vi "PH_AWG-510.ProcCases.vi"(0 "i ref in":refnum<vi>, 1 "selector":string, 2 "Data":T1, 3 "call cluster":T2={"Object"="", "Selector"="", "CallType"=enum."synchronous", "Async Object"="", "Async Selector"="", "Data Descriptor"="", "Data"=[], "Error #"=0, "Expire"=0}, 5 "error in":errorcluster) -> (14 "i ref out":refnum<vi>, 17 "answer cluster":T2={"Object"="", "Selector"="", "CallType"=enum."synchronous", "Async Object"="", "Async Selector"="", "Data Descriptor"="", "Data"=[], "Error #"=0, "Expire"=0}, 19 "error out":errorcluster)   [LabVIEW 2014, in "PH_AWG-510.lvlib"]
doc: "This method is called by a process from within the default case in the event loop. The methods of a class that are linked to events will be called from THIS method. Add your code here."
uses:
  PH_AWG-510.lvlib
  CS_Core/CSSystem/CoreDefs/CoreDefs.call_type.ctl
  CS_Core/BaseProcess/BaseProcess.descriptor string definition.ctl
  CS_Core/CSSystem/CoreDefs/CoreDefs.rawDataType.ctl
  PH_AWG-510.Trigger Settings.ctl
  CS_Core/CSSystem/CoreLib/CoreLib.byte array 2 short.vi
  CS_Core/CSSystem/CoreLib/CoreLib.string 2 byte array.vi
  CS_Core/CSSystem/CoreLib/CoreLib.byte array 2 string.vi
  CS_Core/CSSystem/CoreLib/CoreLib.byte array 2 double.vi
  CS_Core/CSSystem/CoreLib/CoreLib.lvlib
  CS_Core/BaseProcess/BaseProcess.lvlib
  CS_Core/CAEObj/CAEObj.lvlib
  PH_Basics/PH_PSDBWriter/PH_PSDBWriter.lvlib
  instr.lib/awg510/Tektronix AWG510.lvlib
  PH_Basics/PH_Common/PH_Common.lvlib
  PH_Basics/PH_StatusHandler/PH_StatusHandler.lvlib
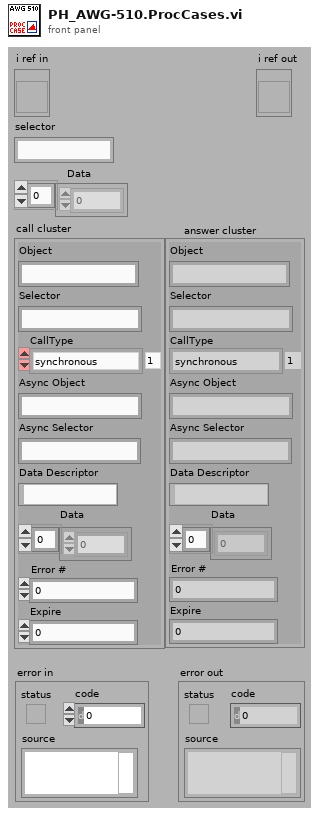
[diagram p1: front panel]
types:
  T1 = typedef "CoreDefs.rawDataType.ctl" = i8[]
  T2 = typedef "CoreDefs.call_type.ctl" = cluster{"Object":string, "Selector":string, "CallType":enum16{"simple", "synchronous", "asynchronous"}, "Async Object":string, "Async Selector":string, "Data Descriptor":T3, "Data":T1, "Error #":i32, "Expire":u32}
  T3 = typedef "BaseProcess.lvlib/BaseProcess.descriptor string definition.ctl" = string
  T4 = typedef "PH_AWG-510.lvlib/PH_AWG-510.Trigger Settings.ctl" = cluster{"Mode":enum16{"Continuous", "Triggered", "Gated", "Enhanced"}, "Level (V)":dbl, "External Source":bool}
  T5 = typedef "PH_AWG-510.lvlib/PH_AWG-510.i attribute.ctl" = cluster{"GUI Refs":cluster{"Delete":refnum<vi>, "Trigger Settings":refnum<vi>, "Start Device":refnum<vi>, "Instrument Information":refnum<vi>, "Lock Frontpanel":refnum<vi>, "Waveform Pattern File":refnum<vi>, "Initialize":refnum<vi>, "Output Settings":refnum<vi>}, "Instrument Information":T6, "Initialized?":bool, "Current Settings":cluster{"Trigger":T4, "Output Settings":T7}, "Wanted Settings":cluster{"Trigger":T4, "Output Settings":T7}, "Device frontpanel locked?":bool, "Default File Path":path}
  T6 = typedef "PH_AWG-510.lvlib/PH_AWG-510.Instrument Information Dataset.ctl" = cluster{"VISA resource name":refnum<visa-resource-name>, "Instrument Firmware Revision":string, "Manufacturer":string, "Model":string, "Serial Number":string, "Error Message":string, "Device Status":enum16{"stopped", "wating for trigger", "running", "Failure"}}
  T7 = typedef "PH_AWG-510.lvlib/PH_AWG-510.Output Settings.ctl" = cluster{"Activate Channel":bool, "VPP (V)":dbl, "Clock (Hz)":dbl, "File Name (Device)":string, "#1":u16, "#2":u16, "#3":u16, "#4":u16, "#5":u16, "#6":u16, "#7":u16, "#8":u16, "#9":u16, "#10":u16, "#11":u16, "#12":u16, "#13":u16, "#14":u16, "#15":u16, "#16":u16, "#17":u16, "#18":u16, "#19":u16, "#20":u16, "Offset (V)":dbl}
  T8 = typedef "PH_PSDBWriter.lvlib/PH_PSDBWriter.PHELIX-Subsystems.ctl" = i32
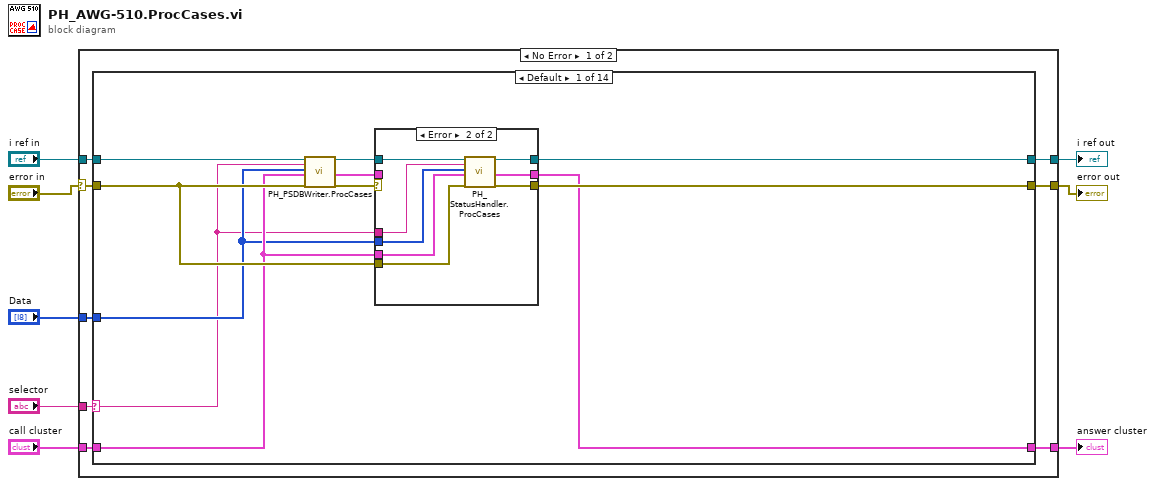
[diagram p0: block diagram]
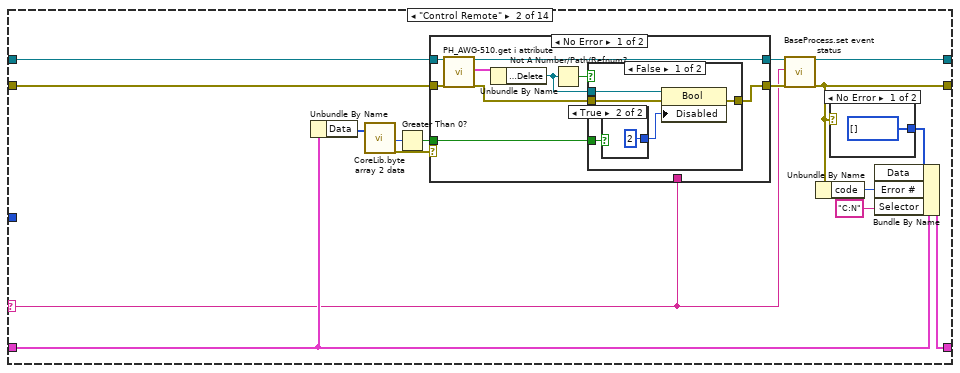
[diagram p3: hidden frame]
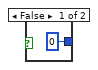
[diagram p4: hidden frame]
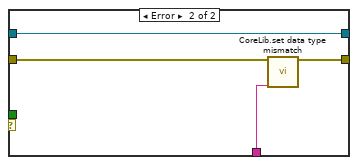
[diagram p6: hidden frame]
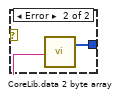
[diagram p7: hidden frame]
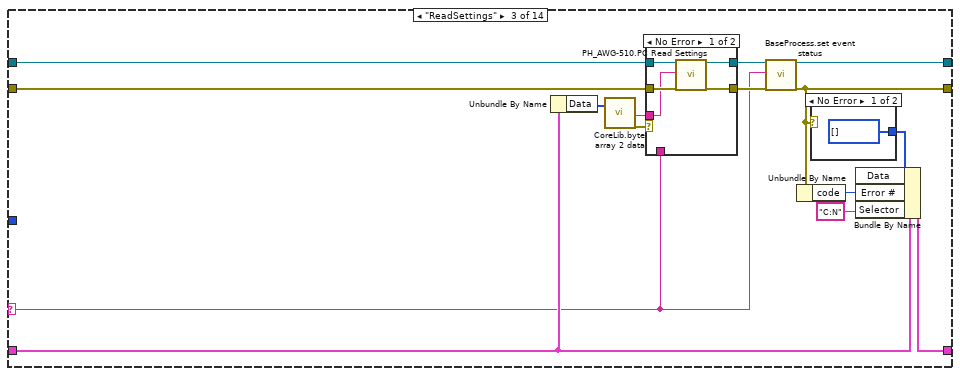
[diagram p8: hidden frame]
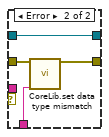
[diagram p9: hidden frame]
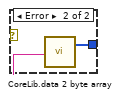
[diagram p10: hidden frame]
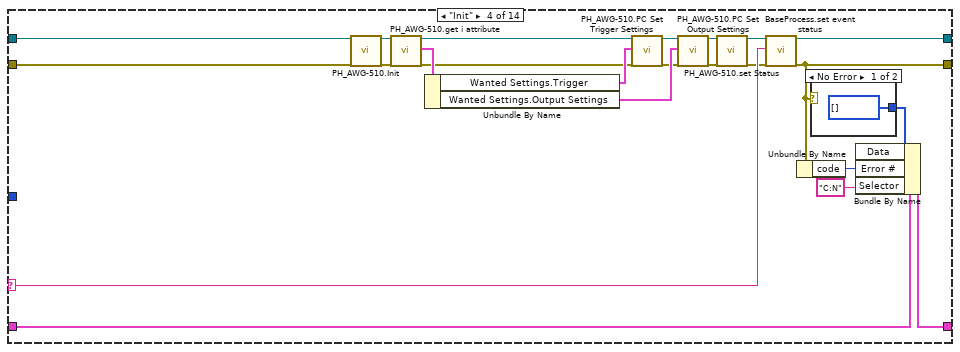
[diagram p11: hidden frame]
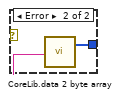
[diagram p12: hidden frame]
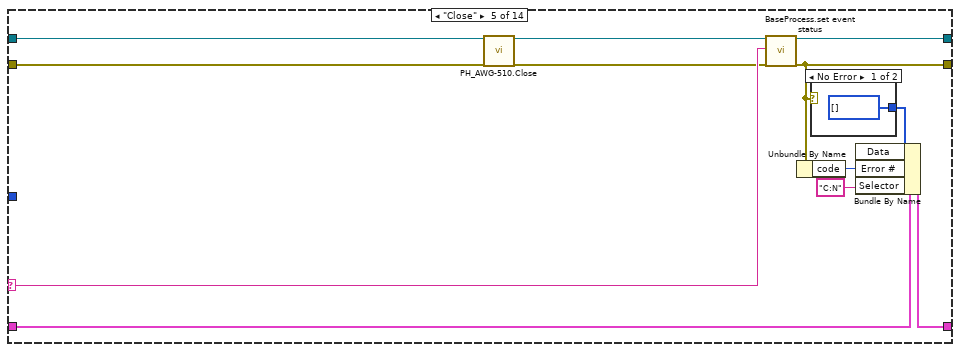
[diagram p13: hidden frame]
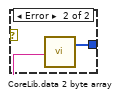
[diagram p14: hidden frame]
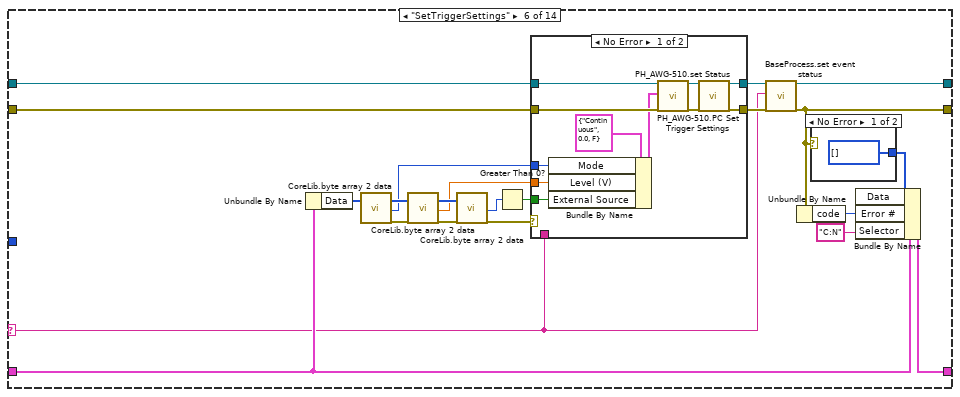
[diagram p15: hidden frame]
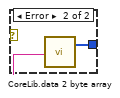
[diagram p17: hidden frame]
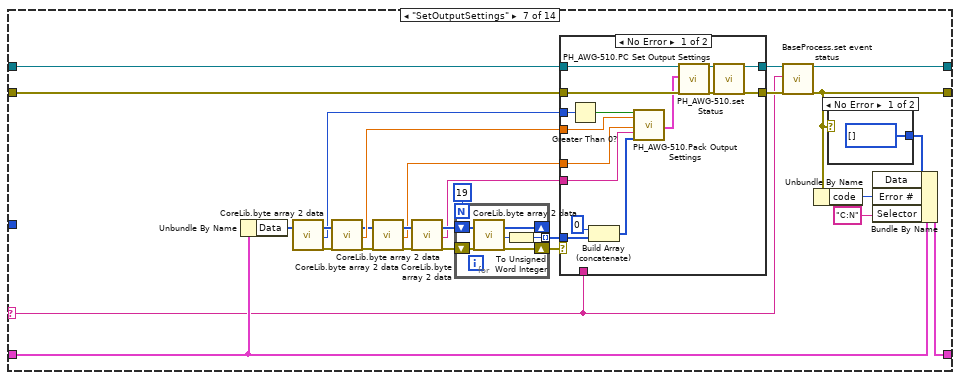
[diagram p18: hidden frame]
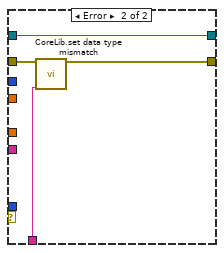
[diagram p19: hidden frame]
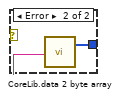
[diagram p20: hidden frame]
diagram:
  n1 = case shown="No Error" "error in" {
    selector: "error in" -> [w9 w513]
    tunnel: "selector" -> [w16 _]
    tunnel: [w15 w514] -> w7
    tunnel: "call cluster" -> [w14 w514]
    tunnel: "i ref in" -> [w13 w515]
    tunnel: [w12 w515] -> w4
    tunnel: [w11 w513] -> w3
    tunnel: "Data" -> [w10 _]
    frame No Error {
      n2 = case shown="Default" w16 {
        selector: w16 -> [w19 w39 w81 w123 w139 w158 w208 w252 w309 w355 w384 w435 w453 w470]
        tunnel: w13 -> [w27 w43 w87 w122 w138 w162 w212 w256 w313 w359 w388 w439 w457 w472]
        tunnel: [w24 w51 w91 w127 w143 w169 w216 w260 w317 w363 w392 w443 w461 w483] -> w12
        tunnel: w14 -> [w21 w40 w83 w124 w140 w159 w209 w253 w310 w356 w385 w436 w454 w480]
        tunnel: [w23 w49 w89 w125 w141 w167 w214 w258 w315 w361 w390 w441 w459 w481] -> w15
        tunnel: w9 -> [w22 w44 w88 w121 w136 w163 w213 w257 w314 w360 w389 w440 w458 w471]
        tunnel: [w26 w50 w90 w126 w142 w168 w215 w259 w316 w362 w391 w442 w460 w482] -> w11
        tunnel: w10 -> [w20 _ _ _ _ _ _ _ _ _ _ _ _ w469]
        frame Default {
          # "In the default case, always call the ProcCase method of the parent class"
          n3 = call "PH_PSDBWriter.ProcCases.vi"("i ref in"=w27, "selector"=w19, "Data"=w20, "call cluster"=w21, "error in"=w22) -> ("i ref out"=w25:refnum<vi>, "answer cluster"=w17:T2, "error out"=w18:errorcluster)  [unwired: 12 in]
          n4 = case shown="Error" w18 {
            selector: w18 -> [w28 _]
            tunnel: [w28 w38] -> w26
            tunnel: w25 -> [w30 w37]
            tunnel: [w30 w36] -> w24
            tunnel: [w29 w35] -> w23
            tunnel: w22 -> [_ w34]
            tunnel: w21 -> [_ w33]
            tunnel: w20 -> [_ w32]
            tunnel: w19 -> [_ w31]
            tunnel: w17 -> [w29 _]
            frame No Error {
            }
            frame Error {
              n5 = call "PH_StatusHandler.ProcCases.vi"("i ref in"=w37, "selector"=w31, "Data"=w32, "call cluster"=w33, "error in (no error)"=w34) -> ("i ref out"=w36:refnum<vi>, "answer cluster"=w35:T2, "error out"=w38:errorcluster)  [unwired: 12 in]
            }
          }
        }
        frame "Control Remote" {
          n6 = Unbundle By Name(w40) -> ("Data"=w45:T1)
          n7 = call-poly "CoreLib.byte array 2 data.vi"("byteArray"=w45) -> ("i16"=w46:i16, "error out"=w48:errorcluster)  [unwired: 16 in, 1 out]
          n8 = Greater Than 0?(x=w46) -> (x > 0?=w47:bool)
          n9 = case shown="No Error" w48 {
            tunnel: [w57 w75] -> w42
            tunnel: w43 -> [w63 w75]
            tunnel: w44 -> [w62 w74]
            tunnel: [w58 w73] -> w41
            tunnel: w39 -> [_ w72]
            tunnel: w47 -> [w59 _]
            frame No Error {
              n10 = call "PH_AWG-510.get i attribute.vi"("i ref in"=w63, "error in (no error)"=w62) -> ("i ref out"=w57:refnum<vi>, "i attribute"=w61:T5, "error out"=w60:errorcluster)  [unwired: 15 in]
              n11 = Unbundle By Name(w61) -> ("GUI Refs.Delete"=w56:refnum<vi>)
              n12 = Not A Number/Path/Refnum?(number/path/refnum=w56) -> (NaN/Path/Refnum?=w55:bool)
              n13 = case shown="False" w55 {
                tunnel: w56 -> [w68 _]
                tunnel: w60 -> [w67 w71]
                tunnel: [w66 w71] -> w58
                tunnel: w59 -> [w65 _]
                frame False {
                  n14 = case shown="True" w65 {
                    tunnel: [0 2] -> w64
                    frame False {
                    }
                    frame True {
                    }
                  }
                  n15 = property class="Bool"(reference=w68, error in=w67, "Disabled"=w64) -> (error out=w66:errorcluster)  [unwired: 1 out]
                }
                frame True {
                }
              }
            }
            frame Error {
              n16 = call "CoreLib.set data type mismatch.vi"("error in (no error)"=w74, "error source"=w72) -> ("error out"=w73:errorcluster)  [unwired: 17 in]
            }
          }
          n17 = call "BaseProcess.set event status.vi"("i ref in"=w42, "EventStatus"=w39, "error in (no error)"=w41) -> ("i ref out"=w51:refnum<vi>, "error out"=w50:errorcluster)  [unwired: 14 in, 1 out]
          n18 = Unbundle By Name(w50) -> ("code"=w54:i32)
          n19 = case shown="No Error" w50 {
            selector: w50 -> [_ w79]
            tunnel: [T1 [] ("byteArray out") w77] -> w53
            frame No Error {
            }
            frame Error {
              n20 = Unbundle By Name(w79) -> ("source"=w78:string)
              n21 = call-poly "CoreLib.data 2 byte array.vi"("string"=w78) -> ("byteArray out"=w77:T1)  [unwired: 18 in]
            }
          }
          n22 = Bundle By Name(cluster=w40, "Data"=w53, "Error #"=w54, "Selector"="C:N") -> (w49:T2)
        }
        frame "ReadSettings" {
          n23 = Unbundle By Name(w83) -> ("Data"=w84:T1)
          n24 = call-poly "CoreLib.byte array 2 data.vi"("byteArray"=w84) -> ("string"=w80:string, "error out"=w82:errorcluster)  [unwired: 16 in, 1 out]
          n25 = case shown="No Error" w82 {
            tunnel: w88 -> [w96 w102]
            tunnel: w87 -> [w99 w100]
            tunnel: [w98 w100] -> w86
            tunnel: [w97 w101] -> w85
            tunnel: w80 -> [w95 _]
            tunnel: w81 -> [_ w103]
            frame No Error {
              n26 = call "PH_AWG-510.PC Read Settings.vi"("VI in"=w99, "File"=w95, "error in (no error)"=w96) -> ("VI out"=w98:refnum<vi>, "error out"=w97:errorcluster)  [unwired: 15 in]
            }
            frame Error {
              n27 = call "CoreLib.set data type mismatch.vi"("error in (no error)"=w102, "error source"=w103) -> ("error out"=w101:errorcluster)  [unwired: 17 in]
            }
          }
          n28 = call "BaseProcess.set event status.vi"("i ref in"=w86, "EventStatus"=w81, "error in (no error)"=w85) -> ("i ref out"=w91:refnum<vi>, "error out"=w90:errorcluster)  [unwired: 14 in, 1 out]
          n29 = Unbundle By Name(w90) -> ("code"=w94:i32)
          n30 = case shown="No Error" w90 {
            selector: w90 -> [_ w107]
            tunnel: [T1 [] ("byteArray out") w105] -> w93
            frame No Error {
            }
            frame Error {
              n31 = Unbundle By Name(w107) -> ("source"=w106:string)
              n32 = call-poly "CoreLib.data 2 byte array.vi"("string"=w106) -> ("byteArray out"=w105:T1)  [unwired: 18 in]
            }
          }
          n33 = Bundle By Name(cluster=w83, "Data"=w93, "Error #"=w94, "Selector"="C:N") -> (w89:T2)
        }
        frame "Init" {
          n34 = call "PH_AWG-510.Init.vi"("VI in"=w122, "error in (no error)"=w121) -> ("VI out"=w111:refnum<vi>, "error out"=w109:errorcluster)  [unwired: 16 in]
          n35 = call "PH_AWG-510.get i attribute.vi"("i ref in"=w111, "error in (no error)"=w109) -> ("i ref out"=w114:refnum<vi>, "i attribute"=w115:T5, "error out"=w112:errorcluster)  [unwired: 15 in]
          n36 = Unbundle By Name(w115) -> ("Wanted Settings.Trigger"=w116:T4, "Wanted Settings.Output Settings"=w118:T7)
          n37 = call "PH_AWG-510.PC Set Trigger Settings.vi"("VI in"=w114, "Wanted Trigger Settings"=w116, "error in (no error)"=w112) -> ("VI out"=w117:refnum<vi>, "error out"=w113:errorcluster)  [unwired: 15 in]
          n38 = call "PH_AWG-510.PC Set Output Settings.vi"("VI in"=w117, "Wanted Output Settings"=w118, "error in (no error)"=w113) -> ("VI out"=w110:refnum<vi>, "error out"=w108:errorcluster)  [unwired: 15 in]
          n39 = call "PH_AWG-510.set Status.vi"("i ref in"=w110, "error in"=w108) -> ("i ref out"=w120:refnum<vi>, "error out"=w119:errorcluster)  [unwired: 16 in]
          n40 = call "BaseProcess.set event status.vi"("i ref in"=w120, "EventStatus"=w123, "error in (no error)"=w119) -> ("i ref out"=w127:refnum<vi>, "error out"=w126:errorcluster)  [unwired: 14 in, 1 out]
          n41 = Unbundle By Name(w126) -> ("code"=w130:i32)
          n42 = case shown="No Error" w126 {
            selector: w126 -> [_ w134]
            tunnel: [T1 [] ("byteArray out") w132] -> w129
            frame No Error {
            }
            frame Error {
              n43 = Unbundle By Name(w134) -> ("source"=w133:string)
              n44 = call-poly "CoreLib.data 2 byte array.vi"("string"=w133) -> ("byteArray out"=w132:T1)  [unwired: 18 in]
            }
          }
          n45 = Bundle By Name(cluster=w124, "Data"=w129, "Error #"=w130, "Selector"="C:N") -> (w125:T2)
        }
        frame "Close" {
          n46 = call "PH_AWG-510.Close.vi"("VI in"=w138, "error in (no error)"=w136) -> ("VI out"=w137:refnum<vi>, "error out"=w135:errorcluster)  [unwired: 16 in]
          n47 = call "BaseProcess.set event status.vi"("i ref in"=w137, "EventStatus"=w139, "error in (no error)"=w135) -> ("i ref out"=w143:refnum<vi>, "error out"=w142:errorcluster)  [unwired: 14 in, 1 out]
          n48 = Unbundle By Name(w142) -> ("code"=w146:i32)
          n49 = case shown="No Error" w142 {
            selector: w142 -> [_ w150]
            tunnel: [T1 [] ("byteArray out") w148] -> w145
            frame No Error {
            }
            frame Error {
              n50 = Unbundle By Name(w150) -> ("source"=w149:string)
              n51 = call-poly "CoreLib.data 2 byte array.vi"("string"=w149) -> ("byteArray out"=w148:T1)  [unwired: 18 in]
            }
          }
          n52 = Bundle By Name(cluster=w140, "Data"=w145, "Error #"=w146, "Selector"="C:N") -> (w141:T2)
        }
        frame "SetTriggerSettings" {
          n53 = Unbundle By Name(w159) -> ("Data"=w156:T1)
          n54 = call-poly "CoreLib.byte array 2 data.vi"("byteArray"=w156) -> ("byteArray out"=w157:T1, "i16"=w152:i16, "error out"=w154:errorcluster)  [unwired: 16 in]
          n55 = call-poly "CoreLib.byte array 2 data.vi"("byteArray"=w157, "error in (no error)"=w154) -> ("byteArray out"=w155:T1, "d64"=w151:dbl, "error out"=w153:errorcluster)  [unwired: 15 in]
          n56 = call-poly "CoreLib.byte array 2 data.vi"("byteArray"=w155, "error in (no error)"=w153) -> ("i16"=w164:i16, "error out"=w166:errorcluster)  [unwired: 15 in, 1 out]
          n57 = Greater Than 0?(x=w164) -> (x > 0?=w165:bool)
          n58 = case shown="No Error" w166 {
            tunnel: [w175 w187] -> w161
            tunnel: w162 -> [w183 w187]
            tunnel: w163 -> [w182 w186]
            tunnel: [w173 w185] -> w160
            tunnel: w158 -> [_ w184]
            tunnel: w165 -> [w178 _]
            tunnel: w152 -> [w180 _]
            tunnel: w151 -> [w179 _]
            frame No Error {
              n59 = Bundle By Name(cluster=T4 {"Mode"=enum."Continuous", "Level (V)"=0.0, "External Source"=FALSE} ("Wanted Trigger Settings"), "Mode"=w180, "Level (V)"=w179, "External Source"=w178) -> (w177:T4)
              n60 = call "PH_AWG-510.PC Set Trigger Settings.vi"("VI in"=w183, "Wanted Trigger Settings"=w177, "error in (no error)"=w182) -> ("VI out"=w176:refnum<vi>, "error out"=w174:errorcluster)  [unwired: 15 in]
              n61 = call "PH_AWG-510.set Status.vi"("i ref in"=w176, "error in"=w174) -> ("i ref out"=w175:refnum<vi>, "error out"=w173:errorcluster)  [unwired: 16 in]
            }
            frame Error {
              n62 = call "CoreLib.set data type mismatch.vi"("error in (no error)"=w186, "error source"=w184) -> ("error out"=w185:errorcluster)  [unwired: 17 in]
            }
          }
          n63 = call "BaseProcess.set event status.vi"("i ref in"=w161, "EventStatus"=w158, "error in (no error)"=w160) -> ("i ref out"=w169:refnum<vi>, "error out"=w168:errorcluster)  [unwired: 14 in, 1 out]
          n64 = Unbundle By Name(w168) -> ("code"=w172:i32)
          n65 = case shown="No Error" w168 {
            selector: w168 -> [_ w191]
            tunnel: [T1 [] ("byteArray out") w189] -> w171
            frame No Error {
            }
            frame Error {
              n66 = Unbundle By Name(w191) -> ("source"=w190:string)
              n67 = call-poly "CoreLib.data 2 byte array.vi"("string"=w190) -> ("byteArray out"=w189:T1)  [unwired: 18 in]
            }
          }
          n68 = Bundle By Name(cluster=w159, "Data"=w171, "Error #"=w172, "Selector"="C:N") -> (w167:T2)
        }
        frame "SetOutputSettings" {
          n69 = Unbundle By Name(w209) -> ("Data"=w206:T1)
          n70 = call-poly "CoreLib.byte array 2 data.vi"("byteArray"=w206) -> ("byteArray out"=w207:T1, "i16"=w204:i16, "error out"=w205:errorcluster)  [unwired: 16 in]
          n71 = call-poly "CoreLib.byte array 2 data.vi"("byteArray"=w207, "error in (no error)"=w205) -> ("byteArray out"=w193:T1, "d64"=w203:dbl, "error out"=w192:errorcluster)  [unwired: 15 in]
          n72 = call-poly "CoreLib.byte array 2 data.vi"("byteArray"=w193, "error in (no error)"=w192) -> ("byteArray out"=w201:T1, "d64"=w200:dbl, "error out"=w202:errorcluster)  [unwired: 15 in]
          n73 = call-poly "CoreLib.byte array 2 data.vi"("byteArray"=w201, "error in (no error)"=w202) -> ("byteArray out"=w198:T1, "string"=w196:string, "error out"=w199:errorcluster)  [unwired: 15 in]
          n74 = for {
            N: 19 -> [_]
            tunnel: [w220] -> w197 mode=indexing
            shift-right: [w222] -> w195
            shift-left: w199 -> [w225]
            shift-right: [w221] -> _
            shift-left: w198 -> [w224]
            n75 = call-poly "CoreLib.byte array 2 data.vi"("byteArray"=w224, "error in (no error)"=w225) -> ("byteArray out"=w221:T1, "i16"=w223:i16, "error out"=w222:errorcluster)  [unwired: 15 in]
            n76 = To Unsigned Word Integer(number=w223) -> (unsigned 16bit integer=w220:u16)
          }
          n77 = case shown="No Error" w195 {
            tunnel: [w234 w244] -> w211
            tunnel: w212 -> [w240 w244]
            tunnel: w213 -> [w239 w243]
            tunnel: [w232 w242] -> w210
            tunnel: w208 -> [_ w241]
            tunnel: w196 -> [w229 _]
            tunnel: w204 -> [w238 _]
            tunnel: w203 -> [w237 _]
            tunnel: w200 -> [w230 _]
            tunnel: w197 -> [w228 _]
            frame No Error {
              n78 = Greater Than 0?(x=w238) -> (x > 0?=w231:bool)
              n79 = Build Array (concatenate)(u16 0, w228) -> (w227:u16[])
              n80 = call "PH_AWG-510.Pack Output Settings.vi"("Activate Channel"=w231, "VPP [Volts]"=w237, "Clock [Hz]"=w230, "File Name"=w229, "Waveform Pattern [#1 ... #20]"=w227) -> ("Output Settings"=w236:T7)  [unwired: 14 in]
              n81 = call "PH_AWG-510.PC Set Output Settings.vi"("VI in"=w240, "Wanted Output Settings"=w236, "error in (no error)"=w239) -> ("VI out"=w235:refnum<vi>, "error out"=w233:errorcluster)  [unwired: 15 in]
              n82 = call "PH_AWG-510.set Status.vi"("i ref in"=w235, "error in"=w233) -> ("i ref out"=w234:refnum<vi>, "error out"=w232:errorcluster)  [unwired: 16 in]
            }
            frame Error {
              n83 = call "CoreLib.set data type mismatch.vi"("error in (no error)"=w243, "error source"=w241) -> ("error out"=w242:errorcluster)  [unwired: 17 in]
            }
          }
          n84 = call "BaseProcess.set event status.vi"("i ref in"=w211, "EventStatus"=w208, "error in (no error)"=w210) -> ("i ref out"=w216:refnum<vi>, "error out"=w215:errorcluster)  [unwired: 14 in, 1 out]
          n85 = Unbundle By Name(w215) -> ("code"=w219:i32)
          n86 = case shown="No Error" w215 {
            selector: w215 -> [_ w248]
            tunnel: [T1 [] ("byteArray out") w246] -> w218
            frame No Error {
            }
            frame Error {
              n87 = Unbundle By Name(w248) -> ("source"=w247:string)
              n88 = call-poly "CoreLib.data 2 byte array.vi"("string"=w247) -> ("byteArray out"=w246:T1)  [unwired: 18 in]
            }
          }
          n89 = Bundle By Name(cluster=w209, "Data"=w218, "Error #"=w219, "Selector"="C:N") -> (w214:T2)
        }
        frame "SetWfmFile" {
          n90 = Unbundle By Name(w253) -> ("Data"=w249:T1)
          n91 = call-poly "CoreLib.byte array 2 data.vi"("byteArray"=w249) -> ("string"=w250:string, "error out"=w251:errorcluster)  [unwired: 16 in, 1 out]
          n92 = case shown="No Error" w251 {
            tunnel: [w272 w301] -> w255
            tunnel: w256 -> [w269 w301]
            tunnel: w257 -> [w270 w300]
            tunnel: [w271 w299] -> w254
            tunnel: w252 -> [_ w298]
            tunnel: w250 -> [w264 _]
            frame No Error {
              n93 = case shown="Default" w264 {
                selector: w264 -> [_ w275]
                tunnel: w270 -> [w273 w283]
                tunnel: w269 -> [w274 w282]
                tunnel: [w273 w280] -> w268
                tunnel: [w274 w276] -> w266
                frame "", "N/A" {
                }
                frame Default {
                  n94 = call "PH_AWG-510.get data to modify.vi"("i ref in"=w282, "error in (no error)"=w283) -> ("i ref out"=w281:refnum<vi>, "i attribute"=w277:T5, "timed out"=w278:bool, "error out"=w279:errorcluster)  [unwired: 14 in]
                  n95 = case shown="False" w278 {
                    tunnel: w281 -> [w292 w297]
                    tunnel: [w291 w297] -> w276
                    tunnel: [w290 w296] -> w280
                    tunnel: w275 -> [w284 _]
                    tunnel: w279 -> [w289 w296]
                    tunnel: w277 -> [w288 _]
                    frame False {
                      n96 = Unbundle By Name(w288) -> ("Initialized?"=w286:bool, "Instrument Information.VISA resource name"=w287:refnum<visa-resource-name>)
                      n97 = Bundle By Name(cluster=w288, "Current Settings.Output Settings.File Name (Device)"=w284, "Wanted Settings.Output Settings.File Name (Device)"=w284) -> (w285:T5)
                      n98 = case shown="True" w286 {
                        tunnel: w284 -> [_ w295]
                        tunnel: w289 -> [_ w294]
                        tunnel: w287 -> [_ w293]
                        frame False {
                        }
                        frame True {
                          n99 = call "SelectWfmFile.vi"("VISA resource name"=w293, "File name"=w295, "error in"=w294) -> ()  [unwired: 15 in, 2 out]
                        }
                      }
                      n100 = call "PH_AWG-510.set modified data.vi"("i ref in"=w292, "i attribute"=w285, "error in (no error)"=w289) -> ("i ref out"=w291:refnum<vi>, "error out"=w290:errorcluster)  [unwired: 15 in]
                    }
                    frame True {
                    }
                  }
                }
              }
              n101 = call "PH_AWG-510.PC Get Output Settings.vi"("VI in"=w266, "error in (no error)"=w268) -> ("VI out"=w265:refnum<vi>, "error out"=w267:errorcluster)  [unwired: 16 in]
              n102 = call "PH_AWG-510.set Status.vi"("i ref in"=w265, "error in"=w267) -> ("i ref out"=w272:refnum<vi>, "error out"=w271:errorcluster)  [unwired: 16 in]
            }
            frame Error {
              n103 = call "CoreLib.set data type mismatch.vi"("error in (no error)"=w300, "error source"=w298) -> ("error out"=w299:errorcluster)  [unwired: 17 in]
            }
          }
          n104 = call "BaseProcess.set event status.vi"("i ref in"=w255, "EventStatus"=w252, "error in (no error)"=w254) -> ("i ref out"=w260:refnum<vi>, "error out"=w259:errorcluster)  [unwired: 14 in, 1 out]
          n105 = Unbundle By Name(w259) -> ("code"=w263:i32)
          n106 = case shown="No Error" w259 {
            selector: w259 -> [_ w305]
            tunnel: [T1 [] ("byteArray out") w303] -> w262
            frame No Error {
            }
            frame Error {
              n107 = Unbundle By Name(w305) -> ("source"=w304:string)
              n108 = call-poly "CoreLib.data 2 byte array.vi"("string"=w304) -> ("byteArray out"=w303:T1)  [unwired: 18 in]
            }
          }
          n109 = Bundle By Name(cluster=w253, "Data"=w262, "Error #"=w263, "Selector"="C:N") -> (w258:T2)
        }
        frame "StartDevice" {
          n110 = Unbundle By Name(w310) -> ("Data"=w306:T1)
          n111 = call-poly "CoreLib.byte array 2 data.vi"("byteArray"=w306) -> ("i16"=w307:i16, "error out"=w308:errorcluster)  [unwired: 16 in, 1 out]
          n112 = case shown="No Error" w308 {
            tunnel: [w321 w347] -> w312
            tunnel: w313 -> [w326 w347]
            tunnel: w314 -> [w327 w346]
            tunnel: [w322 w345] -> w311
            tunnel: w309 -> [_ w344]
            tunnel: w307 -> [w325 _]
            frame No Error {
              n113 = flat-sequence {
                tunnel: w327 -> [w336]
                tunnel: w326 -> [w335]
                tunnel: w325 -> [w334]
                tunnel: [w333] -> w324
                tunnel: [w332] -> w323
                tunnel: [w340] -> w322
                tunnel: [w342] -> w321
                tunnel: w324 -> [w343]
                tunnel: w323 -> [w341]
                frame #0 {
                  n114 = call "PH_AWG-510.get i attribute.vi"("i ref in"=w335, "error in (no error)"=w336) -> ("i ref out"=w333:refnum<vi>, "i attribute"=w330:T5, "error out"=w332:errorcluster)  [unwired: 15 in]
                  n115 = Greater Than 0?(x=w334) -> (x > 0?=w331:bool)
                  n116 = Unbundle By Name(w330) -> ("Initialized?"=w328:bool, "Instrument Information.VISA resource name"=w329:refnum<visa-resource-name>)
                  n117 = case shown="True" w328 {
                    tunnel: w331 -> [_ w338]
                    tunnel: w332 -> [_ w339]
                    tunnel: w329 -> [_ w337]
                    frame False {
                    }
                    frame True {
                      n118 = call "SetRun.vi"("VISA resource name"=w337, "State"=w338, "error in"=w339) -> ()  [unwired: 15 in, 2 out]
                    }
                  }
                }
                frame #1 {
                  n119 = call "PH_AWG-510.set Status.vi"("i ref in"=w343, "error in"=w341) -> ("i ref out"=w342:refnum<vi>, "error out"=w340:errorcluster)  [unwired: 16 in]
                }
              }
            }
            frame Error {
              n120 = call "CoreLib.set data type mismatch.vi"("error in (no error)"=w346, "error source"=w344) -> ("error out"=w345:errorcluster)  [unwired: 17 in]
            }
          }
          n121 = call "BaseProcess.set event status.vi"("i ref in"=w312, "EventStatus"=w309, "error in (no error)"=w311) -> ("i ref out"=w317:refnum<vi>, "error out"=w316:errorcluster)  [unwired: 14 in, 1 out]
          n122 = Unbundle By Name(w316) -> ("code"=w320:i32)
          n123 = case shown="No Error" w316 {
            selector: w316 -> [_ w351]
            tunnel: [T1 [] ("byteArray out") w349] -> w319
            frame No Error {
            }
            frame Error {
              n124 = Unbundle By Name(w351) -> ("source"=w350:string)
              n125 = call-poly "CoreLib.data 2 byte array.vi"("string"=w350) -> ("byteArray out"=w349:T1)  [unwired: 18 in]
            }
          }
          n126 = Bundle By Name(cluster=w310, "Data"=w319, "Error #"=w320, "Selector"="C:N") -> (w315:T2)
        }
        frame "SetExpMode" {
          n127 = Unbundle By Name(w356) -> ("Data"=w352:T1)
          n128 = call-poly "CoreLib.byte array 2 data.vi"("byteArray"=w352) -> ("i16"=w353:i16, "error out"=w354:errorcluster)  [unwired: 16 in, 1 out]
          n129 = case shown="Error" w354 {
            tunnel: [w370 w376] -> w358
            tunnel: w359 -> [w368 w376]
            tunnel: w360 -> [w369 w375]
            tunnel: [w371 w374] -> w357
            tunnel: w355 -> [_ w373]
            tunnel: w353 -> [w372 _]
            frame No Error {
              n130 = Greater Than 0?(x=w372) -> (x > 0?=w367:bool)
              n131 = call "PH_AWG-510.PC Set Expert Mode.vi"("VI in"=w368, "Expert Mode"=w367, "error in (no error)"=w369) -> ("VI out"=w370:refnum<vi>, "error out"=w371:errorcluster)  [unwired: 15 in]
            }
            frame Error {
              n132 = call "CoreLib.set data type mismatch.vi"("error in (no error)"=w375, "error source"=w373) -> ("error out"=w374:errorcluster)  [unwired: 17 in]
            }
          }
          n133 = call "BaseProcess.set event status.vi"("i ref in"=w358, "EventStatus"=w355, "error in (no error)"=w357) -> ("i ref out"=w363:refnum<vi>, "error out"=w362:errorcluster)  [unwired: 14 in, 1 out]
          n134 = Unbundle By Name(w362) -> ("code"=w366:i32)
          n135 = case shown="No Error" w362 {
            selector: w362 -> [_ w380]
            tunnel: [T1 [] ("byteArray out") w378] -> w365
            frame No Error {
            }
            frame Error {
              n136 = Unbundle By Name(w380) -> ("source"=w379:string)
              n137 = call-poly "CoreLib.data 2 byte array.vi"("string"=w379) -> ("byteArray out"=w378:T1)  [unwired: 18 in]
            }
          }
          n138 = Bundle By Name(cluster=w356, "Data"=w365, "Error #"=w366, "Selector"="C:N") -> (w361:T2)
        }
        frame "LockDevice" {
          n139 = Unbundle By Name(w385) -> ("Data"=w381:T1)
          n140 = call-poly "CoreLib.byte array 2 data.vi"("byteArray"=w381) -> ("i16"=w382:i16, "error out"=w383:errorcluster)  [unwired: 16 in, 1 out]
          n141 = case shown="No Error" w383 {
            tunnel: [w402 w428] -> w387
            tunnel: w388 -> [w406 w428]
            tunnel: w389 -> [w407 w427]
            tunnel: [w403 w426] -> w386
            tunnel: w384 -> [_ w425]
            tunnel: w382 -> [w405 _]
            frame No Error {
              n142 = Greater Than 0?(x=w405) -> (x > 0?=w397:bool)
              n143 = call "PH_AWG-510.get data to modify.vi"("i ref in"=w406, "error in (no error)"=w407) -> ("i ref out"=w400:refnum<vi>, "i attribute"=w398:T5, "timed out"=w396:bool, "error out"=w404:errorcluster)  [unwired: 14 in]
              n144 = case shown="False" w396 {
                tunnel: w404 -> [w419 w423]
                tunnel: [w417 w423] -> w401
                tunnel: w400 -> [w416 w424]
                tunnel: [w415 w424] -> w399
                tunnel: w398 -> [w414 _]
                tunnel: w397 -> [w410 _]
                frame False {
                  n145 = Unbundle By Name(w414) -> ("GUI Refs.Lock Frontpanel"=w411:refnum<vi>, "Initialized?"=w409:bool, "Instrument Information.VISA resource name"=w418:refnum<visa-resource-name>)
                  n146 = Select(t=w410, s=w409, f=w409) -> (s? t:f=w408:bool)
                  n147 = Bundle By Name(cluster=w414, "Device frontpanel locked?"=w408) -> (w413:T5)
                  n148 = call "PH_GUI.set boolean GUI object.vi"("Boolean Knob GUI Ref"=w411, "Value"=w408, "error in (no error)"=w419) -> ("error out"=w412:errorcluster)  [unwired: 16 in]
                  n149 = case shown="True" w409 {
                    tunnel: w410 -> [_ w421]
                    tunnel: w419 -> [_ w422]
                    tunnel: w418 -> [_ w420]
                    frame False {
                    }
                    frame True {
                      n150 = call "SetPanelLock.vi"("VISA resource name"=w420, "Status (Lock)"=w421, "error in"=w422) -> ()  [unwired: 15 in, 2 out]
                    }
                  }
                  n151 = call "PH_AWG-510.set modified data.vi"("i ref in"=w416, "i attribute"=w413, "error in (no error)"=w412) -> ("i ref out"=w415:refnum<vi>, "error out"=w417:errorcluster)  [unwired: 15 in]
                }
                frame True {
                }
              }
              n152 = call "PH_AWG-510.set Status.vi"("i ref in"=w399, "error in"=w401) -> ("i ref out"=w402:refnum<vi>, "error out"=w403:errorcluster)  [unwired: 16 in]
            }
            frame Error {
              n153 = call "CoreLib.set data type mismatch.vi"("error in (no error)"=w427, "error source"=w425) -> ("error out"=w426:errorcluster)  [unwired: 17 in]
            }
          }
          n154 = call "BaseProcess.set event status.vi"("i ref in"=w387, "EventStatus"=w384, "error in (no error)"=w386) -> ("i ref out"=w392:refnum<vi>, "error out"=w391:errorcluster)  [unwired: 14 in, 1 out]
          n155 = Unbundle By Name(w391) -> ("code"=w395:i32)
          n156 = case shown="No Error" w391 {
            selector: w391 -> [_ w432]
            tunnel: [T1 [] ("byteArray out") w430] -> w394
            frame No Error {
            }
            frame Error {
              n157 = Unbundle By Name(w432) -> ("source"=w431:string)
              n158 = call-poly "CoreLib.data 2 byte array.vi"("string"=w431) -> ("byteArray out"=w430:T1)  [unwired: 18 in]
            }
          }
          n159 = Bundle By Name(cluster=w385, "Data"=w394, "Error #"=w395, "Selector"="C:N") -> (w390:T2)
        }
        frame "GetTriggerSettings" {
          n160 = call "PH_AWG-510.PC Get Trigger Settings.vi"("VI in"=w439, "error in (no error)"=w440) -> ("VI out"=w434:refnum<vi>, "error out"=w433:errorcluster)  [unwired: 16 in]
          n161 = call "PH_AWG-510.set Status.vi"("i ref in"=w434, "error in"=w433) -> ("i ref out"=w438:refnum<vi>, "error out"=w437:errorcluster)  [unwired: 16 in]
          n162 = call "BaseProcess.set event status.vi"("i ref in"=w438, "EventStatus"=w435, "error in (no error)"=w437) -> ("i ref out"=w443:refnum<vi>, "error out"=w442:errorcluster)  [unwired: 14 in, 1 out]
          n163 = Unbundle By Name(w442) -> ("code"=w446:i32)
          n164 = case shown="No Error" w442 {
            selector: w442 -> [_ w450]
            tunnel: [T1 [] ("byteArray out") w448] -> w445
            frame No Error {
            }
            frame Error {
              n165 = Unbundle By Name(w450) -> ("source"=w449:string)
              n166 = call-poly "CoreLib.data 2 byte array.vi"("string"=w449) -> ("byteArray out"=w448:T1)  [unwired: 18 in]
            }
          }
          n167 = Bundle By Name(cluster=w436, "Data"=w445, "Error #"=w446, "Selector"="C:N") -> (w441:T2)
        }
        frame "GetOutputSettings" {
          n168 = call "PH_AWG-510.PC Get Output Settings.vi"("VI in"=w457, "error in (no error)"=w458) -> ("VI out"=w452:refnum<vi>, "error out"=w451:errorcluster)  [unwired: 16 in]
          n169 = call "PH_AWG-510.set Status.vi"("i ref in"=w452, "error in"=w451) -> ("i ref out"=w456:refnum<vi>, "error out"=w455:errorcluster)  [unwired: 16 in]
          n170 = call "BaseProcess.set event status.vi"("i ref in"=w456, "EventStatus"=w453, "error in (no error)"=w455) -> ("i ref out"=w461:refnum<vi>, "error out"=w460:errorcluster)  [unwired: 14 in, 1 out]
          n171 = Unbundle By Name(w460) -> ("code"=w464:i32)
          n172 = case shown="No Error" w460 {
            selector: w460 -> [_ w468]
            tunnel: [T1 [] ("byteArray out") w466] -> w463
            frame No Error {
            }
            frame Error {
              n173 = Unbundle By Name(w468) -> ("source"=w467:string)
              n174 = call-poly "CoreLib.data 2 byte array.vi"("string"=w467) -> ("byteArray out"=w466:T1)  [unwired: 18 in]
            }
          }
          n175 = Bundle By Name(cluster=w454, "Data"=w463, "Error #"=w464, "Selector"="C:N") -> (w459:T2)
        }
        frame "_set_PSDB_Data" {
          n176 = call "CAEObj.unfold trend data.vi"("i ref in"=w472, "raw trend data"=w469) -> ("quality"=w475:i32, "no link"=w478:bool, "data"=w476:i8[], "typeDescriptor"=w477:string, "error out"=w479:errorcluster)  [unwired: 9 in, 4 out]
          n177 = case shown="No Error" w479 {
            tunnel: w471 -> [w498 w508]
            tunnel: [w497 w507] -> w474
            tunnel: [w496 w508] -> w473
            tunnel: w472 -> [w494 w507]
            tunnel: w478 -> [w487 _]
            tunnel: w477 -> [w489 _]
            tunnel: w476 -> [w490 _]
            tunnel: w475 -> [w488 _]
            frame No Error {
              n178 = call "PH_PSDBWriter.get Subsystem DIM Service.vi"("no link"=w487, "typeDescriptor"=w489, "data"=w490, "quality"=w488) -> ("PHELIX Subsystems"=w491:T8)
              n179 = call "PH_PSDBWriter.check PSDB writing condition.vi"("i ref in"=w494, "wanted Subsystem"=w491, "error IO"=w498) -> ("i ref out"=w493:refnum<vi>, "write PSDB?"=w492:bool, "error out"=w495:errorcluster)  [unwired: 14 in]
              n180 = case shown="True" w492 {
                tunnel: w495 -> [w499 w506]
                tunnel: [w500 w503] -> w497
                tunnel: [w499 w501] -> w496
                tunnel: w493 -> [w500 w505]
                frame False {
                }
                frame True {
                  n181 = call "PH_AWG-510.PC Write PSDB.vi"("i ref in"=w505, "error IO"=w506) -> ("i ref out"=w504:refnum<vi>, "error out"=w502:errorcluster)  [unwired: 16 in]
                  n182 = call "PH_PSDBWriter.evt call write PSDB.vi"("i ref in"=w504, "error in (no error)"=w502) -> ("i ref out"=w503:refnum<vi>, "error out"=w501:errorcluster)  [unwired: 16 in]
                }
              }
            }
            frame Error {
            }
          }
          n183 = call "BaseProcess.set event status.vi"("i ref in"=w474, "EventStatus"=w470, "error in (no error)"=w473) -> ("i ref out"=w483:refnum<vi>, "error out"=w482:errorcluster)  [unwired: 14 in, 1 out]
          n184 = Unbundle By Name(w482) -> ("code"=w486:i32)
          n185 = case shown="No Error" w482 {
            selector: w482 -> [_ w512]
            tunnel: [T1 [] ("byteArray out") w510] -> w485
            frame No Error {
            }
            frame Error {
              n186 = Unbundle By Name(w512) -> ("source"=w511:string)
              n187 = call-poly "CoreLib.data 2 byte array.vi"("string"=w511) -> ("byteArray out"=w510:T1)  [unwired: 18 in]
            }
          }
          n188 = Bundle By Name(cluster=w480, "Data"=w485, "Error #"=w486, "Selector"="C:N") -> (w481:T2)
        }
      }
    }
    frame Error {
    }
  }
  "answer cluster" <- w7
  "i ref out" <- w4
  "error out" <- w3
